vi "TitleString.vi"(8 "error in":errorcluster, 9 "Task":string, 10 "Trial":i32, 11 "Subject":string) -> (0 "error out":errorcluster, 3 "String":string)   [LabVIEW 2020, in "CollectionSupport.lvlib"]
uses:
  CollectionSupport.lvlib
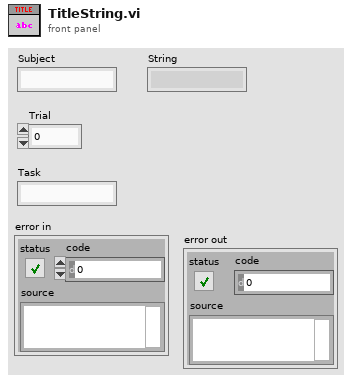
[diagram p1: front panel]
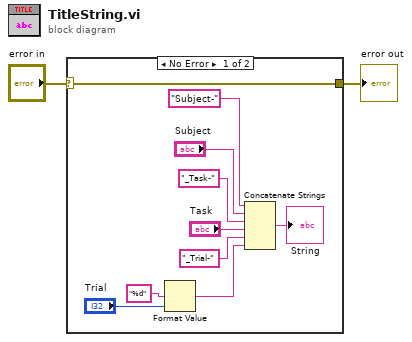
[diagram p0: block diagram]
diagram:
  n1 = case shown="No Error" "error in" {
    selector: "error in" -> [w4 w13]
    tunnel: [w4 w13] -> w1
    frame No Error {
      n2 = Format Value(format string="%d", value (0)="Trial") -> (output string=w11:string)  [unwired: 1 in]
      n3 = Concatenate Strings("Subject-" ("string"), "Subject", "_Task-" ("string"), "Task", "_Trial-" ("string"), w11) -> (→"String":string)
    }
    frame Error {
    }
  }
  "error out" <- w1
